vi "GENser Initialize.vi"(5 "ID Query (T)":bool=TRUE, 6 "Timeout (3 sec)":dbl=3.0 format="%.2f", 7 "Reset (T)":bool=TRUE, 8 "error in (no error)":errorcluster, 9 "BAUD":u16(ring)=3 items=["1200", "2400", "4800", "9600", "19200"], 10 "GEN Addr":i16=6, 11 "VISA name":refnum<visa-resource-name>) -> (0 "error out":errorcluster, 3 "VISA out":refnum<visa-resource-name>)   [LabVIEW 2017]
doc: "This VI uses the serial port specified in \"VISA name\" to send the \"Address\" command to the Genesys power supply. You must run this VI before using any of the instrument driver VIs for this instrument.\n\nYou can optionally reset the instrument by setting the front panel reset control. \nYou can optionally read the instrument identity string and verify ithe instrument can be used with this driver.\n\nThe Timeout is the number of seconds allowed for instrument to respond. The default is 3 seconds."
panel:
  # "Lambda Genesys \n Serial Port\n  DC Power Supplies"
  # "Initialize Instrument\nOpen VISA Port"
  # "Seconds"
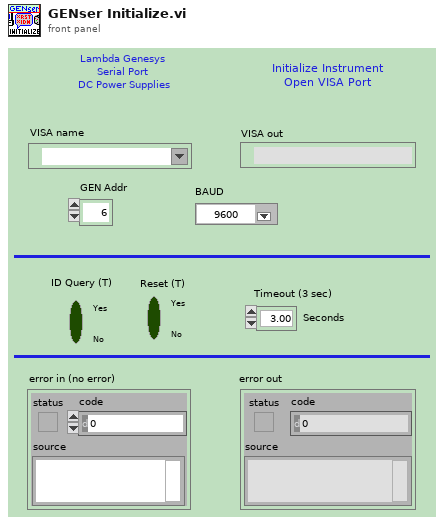
[diagram p1: front panel]
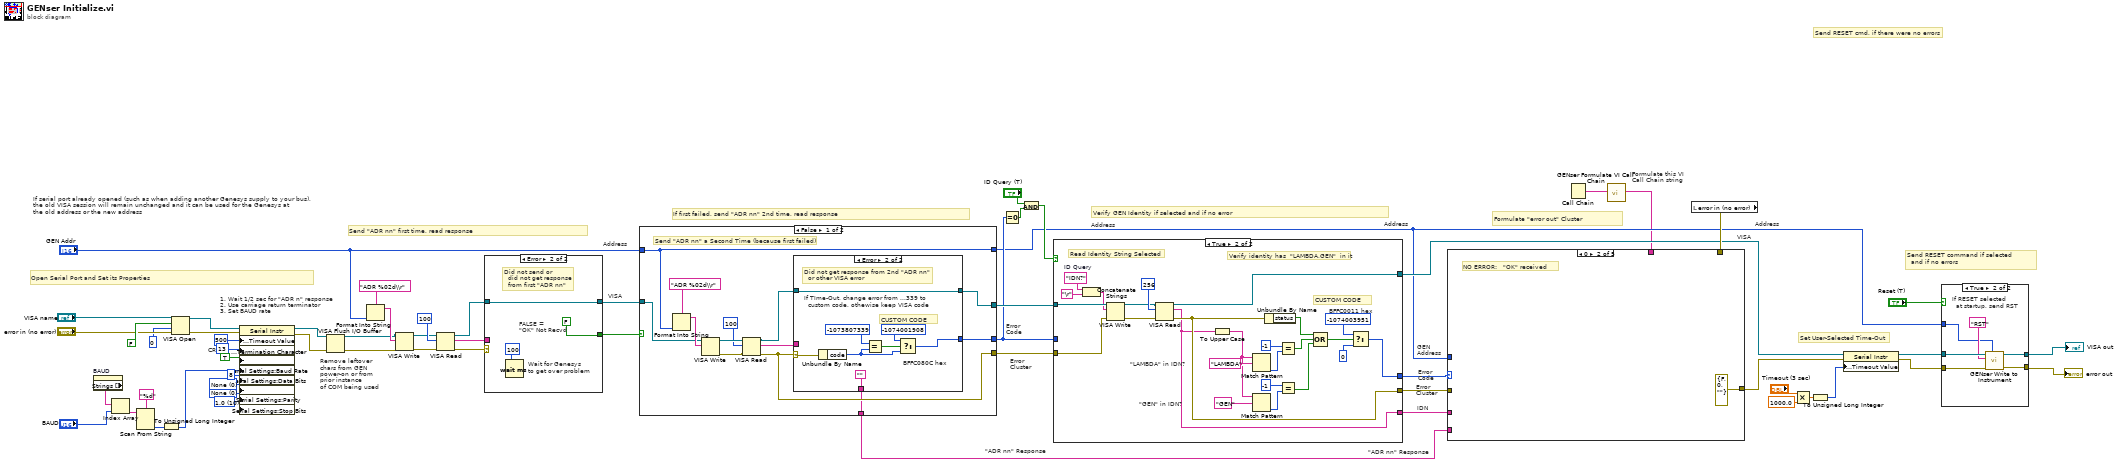
[diagram p0: block diagram]
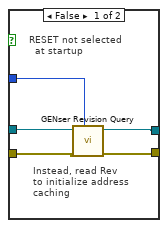
[diagram p2: hidden frame]
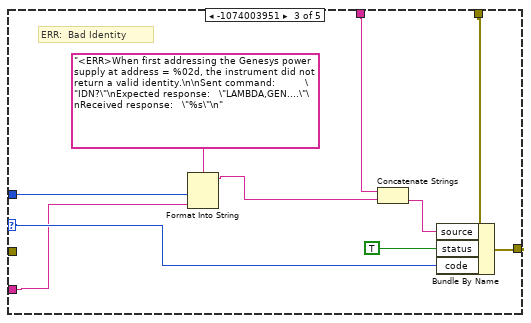
[diagram p4: hidden frame]
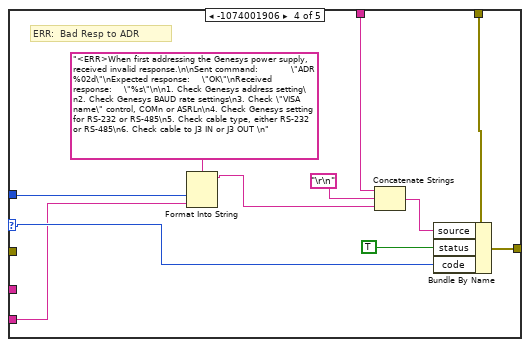
[diagram p5: hidden frame]
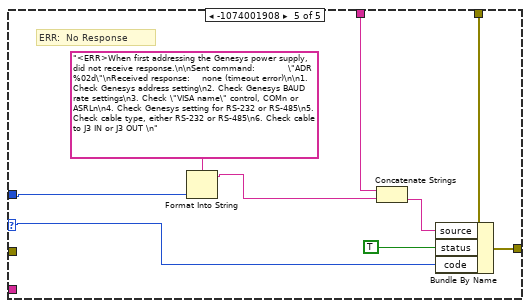
[diagram p6: hidden frame]
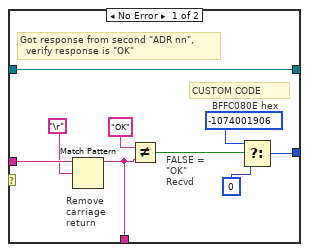
[diagram p7: hidden frame]
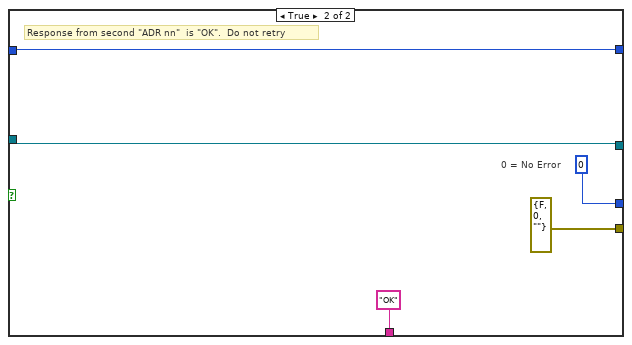
[diagram p8: hidden frame]
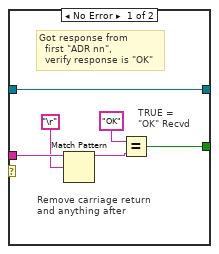
[diagram p9: hidden frame]
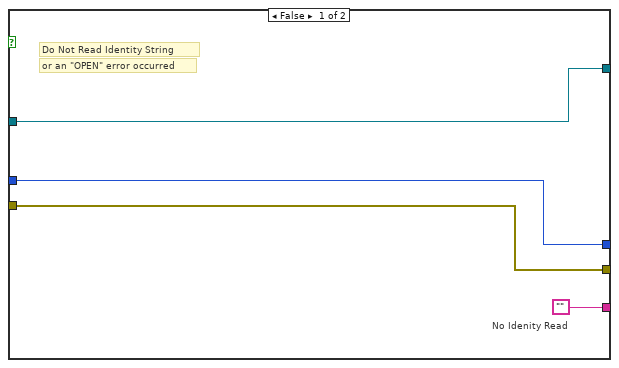
[diagram p10: hidden frame]
diagram:
  w11 = u16 10 items=["1.0"=10, "1.5"=15, "2.0"=20] ("Serial Settings:Serial Stop Bits")
  w12 = u16 0 items=["None", "Odd", "Even", "Mark", "Space"] ("Serial Settings:Serial Parity")
  w13 = u16 0 items=["None", "XON/XOFF", "RTS/CTS", "XON/XOFF & RTS/CTS", "DTR/DSR", "XON/XOFF & DTR/DSR"] ("Serial Settings:Serial Flow Control")
  # "Formulate this VI \nCall Chain string"
  # "Remove leftover\nchars from GEN\npower-on or from\nprior instance\nof COM being used"
  # "CR"
  # "Address"
  # "Send RESET command if selected  \n  and if no errors"
  # "Send RESET cmd, if there were no errors"
  # "VISA"
  # "GEN\nAddress"
  # "Formulate \"error out\" Cluster"
  # "\"ADR nn\" Response"
  # "\"ADR nn\" Response"
  # "IDN"
  # "Error\nCluster"
  # "Address"
  # "Error\nCode"
  # "Verify GEN Identity if selected and if no error"
  # "Error\nCluster"
  # "Error\nCode"
  # "Address"
  # "If first failed, send \"ADR nn\" 2nd time, read response"
  # "VISA"
  # "Address"
  # "Set User-Selected Time-Out"
  # "Send \"ADR nn\" first time, read response"
  # "1. Wait 1/2 sec for \"ADR n\" response\n2. Use carriage return terminator\n3. Set BAUD rate"
  # "Open Serial Port and Set its Properties"
  # "If serial port already opened (such as when adding another Genesys supply to your bus),\nthe old VISA session will remain unchanged and it can be used for the Genesys at \nthe old address or the new address"
  n1 = property on="BAUD" class="Ring (strict)"() -> ("Strings []"=w53:string[])  [unwired: 2 in, 2 out]
  n2 = Index Array(array=w53, index="BAUD") -> (element=w55:string)
  n3 = Scan From String(format string="%d", input string=w55) -> (output 1=w56:i32)  [unwired: 3 in, 3 out]
  n4 = To Unsigned Long Integer(number=w56) -> (unsigned 32bit integer=w57:u32)
  n5 = VISA Open(duplicate session (F)=FALSE, access mode=u32 0, error in (no error)="error in (no error)", VISA resource name="VISA name") -> (VISA resource name=w49:refnum<visa-resource-name>, error out=w50:errorcluster)  [unwired: 1 in]
  n6 = property class="Serial Instr"(reference=w49, error in=w50, "General Settings:Timeout Value"=u32 500, "Message Based Settings:Termination Character"=u8 13, "Message Based Settings:Termination Character Enable"=TRUE, "Serial Settings:Baud Rate"=w57, "Serial Settings:Data Bits"=u16 8 ("Serial Settings:Serial Data Bits"), "Serial Settings:Flow Control"=w13, "Serial Settings:Parity"=w12, "Serial Settings:Stop Bits"=w11) -> (reference out=w10:refnum<visa-resource-name>, error out=w9:errorcluster)
  n7 = VISA Flush I/O Buffer(VISA resource name=w10, error in (no error)=w9) -> (VISA resource name out=w7:refnum<visa-resource-name>, error out=w8:errorcluster)  [unwired: 1 in]
  n8 = Format Into String(format string="ADR %02d\\r", "GEN Addr") -> (resulting string=w40:string)  [unwired: 2 in, 1 out]
  n9 = VISA Write(VISA resource name=w7, write buffer=w40, error in (no error)=w8) -> (VISA resource name out=w41:refnum<visa-resource-name>, error out=w42:errorcluster)  [unwired: 1 out]
  n10 = VISA Read(VISA resource name=w41, byte count=u32 100 ("byte count (0)"), error in (no error)=w42) -> (VISA resource name out=w34:refnum<visa-resource-name>, read buffer=w37:string, error out=w38:errorcluster)  [unwired: 1 out]
  n11 = case shown="Error" w38 {
    tunnel: w37 -> [w63 _]
    tunnel: [w62 FALSE] -> w36
    tunnel: [w61 w66] -> w33
    tunnel: w34 -> [w61 w66]
    frame No Error {
      # "TRUE = \n\"OK\" Recvd"
      # "Remove carriage return\nand anything after"
      # "Got response from \n  first \"ADR nn\",  \n  verify response is \"OK\""
      n12 = Match Pattern(string=w63, regular expression="\r") -> (before substring=w65:string)  [unwired: 1 in, 3 out]
      n13 = Equal?(x="OK" ("regular expression"), y=w65) -> (x = y?=w62:bool)
    }
    frame Error {
      # "FALSE = \n\"OK\" Not Recvd"
      # "Wait for Genesys\nto get over problem"
      # "Did not send or  \n  did not get response  \n  from first \"ADR nn\""
      n14 = Wait (ms)(milliseconds to wait=u32 100) -> ()  [unwired: 1 out]
    }
  }
  n15 = case shown="False" w36 {
    tunnel: w33 -> [w76 w100]
    tunnel: "GEN Addr" -> [w70 w102]
    tunnel: [w73 0 ("code")] -> w25
    tunnel: [w72 errorcluster {"status"=FALSE, "code"=0, "source"=""} ("error IO")] -> w28
    tunnel: [w71 w100] -> w27
    tunnel: [w70 w102] -> w6
    tunnel: [w69 "OK"] -> w22
    frame False {
      # "Send \"ADR nn\" a Second Time (because first failed)"
      n16 = Format Into String(format string="ADR %02d\\r", w70) -> (resulting string=w80:string)  [unwired: 2 in, 1 out]
      n17 = VISA Write(VISA resource name=w76, write buffer=w80) -> (VISA resource name out=w79:refnum<visa-resource-name>, error out=w78:errorcluster)  [unwired: 1 in, 1 out]
      n18 = VISA Read(VISA resource name=w79, byte count=u32 100 ("byte count (0)"), error in (no error)=w78) -> (VISA resource name out=w74:refnum<visa-resource-name>, read buffer=w75:string, error out=w72:errorcluster)  [unwired: 1 out]
      n19 = case shown="Error" w72 {
        selector: w72 -> [_ w97]
        tunnel: w75 -> [w89 _]
        tunnel: [w88 w98] -> w71
        tunnel: w74 -> [w88 w98]
        tunnel: [w84 w92] -> w73
        tunnel: [w83 ""] -> w69
        frame No Error {
          # "CUSTOM CODE"
          # "BFFC080E hex"
          # "FALSE = \n\"OK\" \nRecvd"
          # "Remove \ncarriage\nreturn"
          # "Got response from second \"ADR nn\",  \n  verify response is \"OK\""
          n20 = Match Pattern(string=w89, regular expression="\r") -> (before substring=w83:string)  [unwired: 1 in, 3 out]
          n21 = Not Equal?(x="OK" ("regular expression"), y=w83) -> (x != y?=w87:bool)
          n22 = Select(t=-1074001906, s=w87, f=0) -> (s? t:f=w84:i32)
        }
        frame Error {
          # "BFFC080C hex"
          # "CUSTOM CODE"
          # "If TIme-Out, change error from ...339 to  \n  custom code, othewise keep VISA code"
          # "Did not get response from 2nd \"ADR nn\"  \n  or other VISA error"
          n23 = Unbundle By Name(w97) -> ("code"=w94:i32)
          n24 = Equal?(x=-1073807339 ("code"), y=w94) -> (x = y?=w95:bool)
          n25 = Select(t=-1074001908 ("code"), s=w95, f=w94) -> (s? t:f=w92:i32)
        }
      }
    }
    frame True {
      # "0 = No Error"
      # "Response from second \"ADR nn\"  is \"OK\".  Do not retry"
    }
  }
  n26 = Equal To 0?(x=w25) -> (x = 0?=w31:bool)
  n27 = And(x="ID Query (T)", y=w31) -> (x .and. y?=w29:bool)
  n28 = case shown="True" w29 {
    tunnel: [w106 w113] -> w24
    tunnel: [w107 w130] -> w21
    tunnel: w27 -> [w107 w131]
    tunnel: w28 -> [w106 w132]
    tunnel: w25 -> [w105 _]
    tunnel: [w105 w109] -> w15
    tunnel: ["" w112] -> w23
    frame False {
      # "No Idenity Read"
      # "or an \"OPEN\" error occurred"
      # "Do Not Read Identity String"
    }
    frame True {
      w117 = "IDN?"  # ID Query
      # "CUSTOM CODE"
      # "BFFC0011 hex"
      # "\"GEN\" in IDN?"
      # "\"LAMBDA\" in IDN?"
      # "Verify identity has  \"LAMBDA,GEN\"  in it"
      # "Read Identity String Selected"
      n29 = Concatenate Strings(w117, "\r") -> (w115:string)
      n30 = VISA Write(VISA resource name=w131, write buffer=w115, error in (no error)=w132) -> (VISA resource name out=w111:refnum<visa-resource-name>, error out=w110:errorcluster)  [unwired: 1 out]
      n31 = VISA Read(VISA resource name=w111, byte count=u32 256, error in (no error)=w110) -> (VISA resource name out=w130:refnum<visa-resource-name>, read buffer=w112:string, error out=w113:errorcluster)  [unwired: 1 out]
      n32 = To Upper Case(1:w112) -> (0:w118:string)
      n33 = Match Pattern(string=w118, regular expression="LAMBDA") -> (offset past match=w127:i32)  [unwired: 1 in, 3 out]
      n34 = Match Pattern(string=w118, regular expression="GEN") -> (offset past match=w125:i32)  [unwired: 1 in, 3 out]
      n35 = Unbundle By Name(w113) -> ("status"=w122:bool)
      n36 = Equal?(x=-1, y=w127) -> (x = y?=w121:bool)
      n37 = Equal?(x=-1, y=w125) -> (x = y?=w120:bool)
      n38 = Compound Arithmetic op=OR(w122, w121, w120) -> (w119:bool)
      n39 = Select(t=-1074003951, s=w119, f=0) -> (s? t:f=w109:i32)
    }
  }
  n40 = Call Chain() -> (call chain=w2:string[])
  n41 = call "GENser Formulate VI Call Chain.vi"("Call Chain"=w2) -> ("String Out"=w1:string)  [unwired: 10 in]
  n42 = local read "error in (no error)"() -> (w32:errorcluster)
  n43 = case shown="0" w15 {
    selector: w15 -> [_ _ w139 w149 w157]
    tunnel: w32 -> [_ _ w136 w146 w160]
    tunnel: w6 -> [_ _ w140 w150 w163]
    tunnel: w1 -> [_ _ w137 w147 w161]
    tunnel: [w133 errorcluster {"status"=FALSE, "code"=0, "source"=""} ("error IO") w135 w145 w156] -> w20
    tunnel: w24 -> [w133 _ _ _ _]
    tunnel: w23 -> [_ _ w138 _ _]
    tunnel: w22 -> [_ _ _ w148 _]
    frame -1, Default {
      # "ERR:  Generic VISA"
    }
    frame 0 {
      # "NO ERROR:   \"OK\" received"
    }
    frame -1074003951 {
      # "ERR:  Bad Identity"
      n44 = Format Into String(format string="<ERR>When first addressing the Genesys power supply at address = %02d, the instrument did not return a valid identity.\n\nSent command:          \"IDN?\"\nExpected response:   \"LAMBDA,GEN....\"\nReceived response:   \"%s\"\n" ("Source (VI Name)"), w140, w138) -> (resulting string=w143:string)  [unwired: 2 in, 1 out]
      n45 = Concatenate Strings(w137, w143) -> (w142:string)
      n46 = Bundle By Name(cluster=w136, "source"=w142, "status"=TRUE, "code"=w139) -> (w135:errorcluster)
    }
    frame -1074001906 {
      # "ERR:  Bad Resp to ADR"
      n47 = Format Into String(format string="<ERR>When first addressing the Genesys power supply, received invalid response.\n\nSent command:           \"ADR %02d\"\nExpected response:    \"OK\"\nReceived response:    \"%s\"\n\n1. Check Genesys address setting\n2. Check Genesys BAUD rate settings\n3. Check \"VISA name\" control, COMn or ASRLn\n4. Check Genesys setting for RS-232 or RS-485\n5. Check cable type, either RS-232 or RS-485\n6. Check cable to J3 IN or J3 OUT \n" ("Source (VI Name)"), w150, w148) -> (resulting string=w153:string)  [unwired: 2 in, 1 out]
      n48 = Concatenate Strings(w147, "\r\n", w153) -> (w152:string)
      n49 = Bundle By Name(cluster=w146, "source"=w152, "status"=TRUE, "code"=w149) -> (w145:errorcluster)
    }
    frame -1074001908 {
      # "ERR:  No Response"
      n50 = Format Into String(format string="<ERR>When first addressing the Genesys power supply, did not receive response.\n\nSent command:           \"ADR %02d\"\nReceived response:    none (timeout error)\n\n1. Check Genesys address setting\n2. Check Genesys BAUD rate settings\n3. Check \"VISA name\" control, COMn or ASRLn\n4. Check Genesys setting for RS-232 or RS-485\n5. Check cable type, either RS-232 or RS-485\n6. Check cable to J3 IN or J3 OUT \n" ("Source (VI Name)"), w163) -> (resulting string=w162:string)  [unwired: 2 in, 1 out]
      n51 = Concatenate Strings(w161, w162) -> (w159:string)
      n52 = Bundle By Name(cluster=w160, "source"=w159, "status"=TRUE, "code"=w157) -> (w156:errorcluster)
    }
  }
  n53 = Multiply(x="Timeout (3 sec)", y=1000.0) -> (x*y=w19:dbl)
  n54 = To Unsigned Long Integer(number=w19) -> (unsigned 32bit integer=w3:u32)
  n55 = property class="Serial Instr"(reference=w21, error in=w20, "General Settings:Timeout Value"=w3) -> (reference out=w17:refnum<visa-resource-name>, error out=w16:errorcluster)
  n56 = case shown="True" "Reset (T)" {
    tunnel: [w167 w175] -> w5
    tunnel: [w166 w174] -> w4
    tunnel: w17 -> [w169 w173]
    tunnel: w16 -> [w168 w171]
    tunnel: w6 -> [w165 w170]
    frame False {
      # "Instead, read Rev\nto initialize address\ncaching"
      # "RESET not selected\n  at startup"
      n57 = call "GENser Revision Query.vi"("GEN Addr"=w165, "error"=w168, "VISA"=w169) -> ("error out"=w166:errorcluster, "VISA out"=w167:refnum<visa-resource-name>)  [unwired: 5 in, 2 out]
    }
    frame True {
      # "If RESET selected\n  at startup, send RST"
      n58 = call "GENser Write to Instrument.vi"("GEN Addr"=w170, "error"=w171, "Command"="RST" ("write buffer (\"\")"), "VISA"=w173) -> ("error out"=w174:errorcluster, "VISA out"=w175:refnum<visa-resource-name>)  [unwired: 5 in, 1 out]
    }
  }
  "VISA out" <- w5
  "error out" <- w4
